vi "test.vi"() -> ()   [LabVIEW 2011]
panel:
  in  "d":bool
  in  "z":bool
  out "x .implies. y?":bool
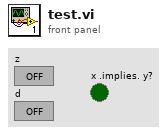
[diagram p1: front panel]
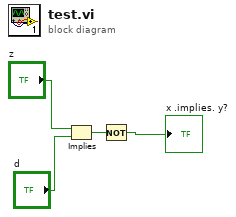
[diagram p0: block diagram]
diagram:
  n1 = Implies(1:"d", 2:"z") -> (0:w4:bool)
  n2 = Not(x=w4) -> (.not. x?=→"x .implies. y?":bool)
